vi "MPB test loop.vi"() -> ()   [LabVIEW 2020]
uses:
  controls/Send Commands.ctl
  src/Main/MPB/controls/MPB Status.ctl
  <vilib>/AKKA/PROVEtech-RBS/PROVEtechRBS.lvlib
panel:
  out "MPB Status":T1 {"InletDCportNegLowRes (VDCportNeg)" format="%.2f"; "HeatgActv (HVIL FB)" format="%.2f"; "InletACportEgy (ACfuseNeg)" format="%.2f"; "InletDCportPosLowRes (VDCportPos)" format="%.2f"; "InletACportFuseLowRes (ACfusePos)" format="%.2f"; "DCbusVoltgUpprHalf" format="%.2f"; "Vac" format="%.2f"; "TrfmrTemp2" format="%.2f"; "TrfmrTemp1" format="%.2f"; "HAPSFltCode" format="%.2f"; "ACCurr4" format="%.2f"; "ACCurr3" format="%.2f"; "ACCurr2" format="%.2f"; "ACCurr1" format="%.2f"; "HAPSCurr" format="%.2f"; "HAPSFltFlag" format="%.2f"; "HAPSVoltgOut" format="%.2f"; "HwFltCode" format="%.2f"; "HwFltFlag" format="%.2f"; "HAPSVoltgIn" format="%.2f"; "BattPortPosFuseLowRes" format="%.2f"; "BattPortNegFuseLowRes" format="%.2f"; "BattPortVoltgLowRes" format="%.2f"; "DCbusVoltg" format="%.2f"; "DCbusVoltgLowrHalf" format="%.2f"; "InletDCportVoltgHiRes" format="%.2f"; "BattPortPower" format="%.2f"; "BattVoltgHiRes" format="%.2f"; "BattCurrDAB2" format="%.2f"; "BattCurrDAB1" format="%.2f"}
  in  "Send Commands":T2
  in  "stop":bool
  # "Other"
  # "AC Port Info"
  # "Battery Port Info"
  # "Fault Info"
  # "1"
  # "2"
  # "3"
  # "4"
  # "5"
  # "6"
  # "7"
  # "DC Bus Info"
  # "HAPS Info"
  # "Temps"
  # "1"
  # "2"
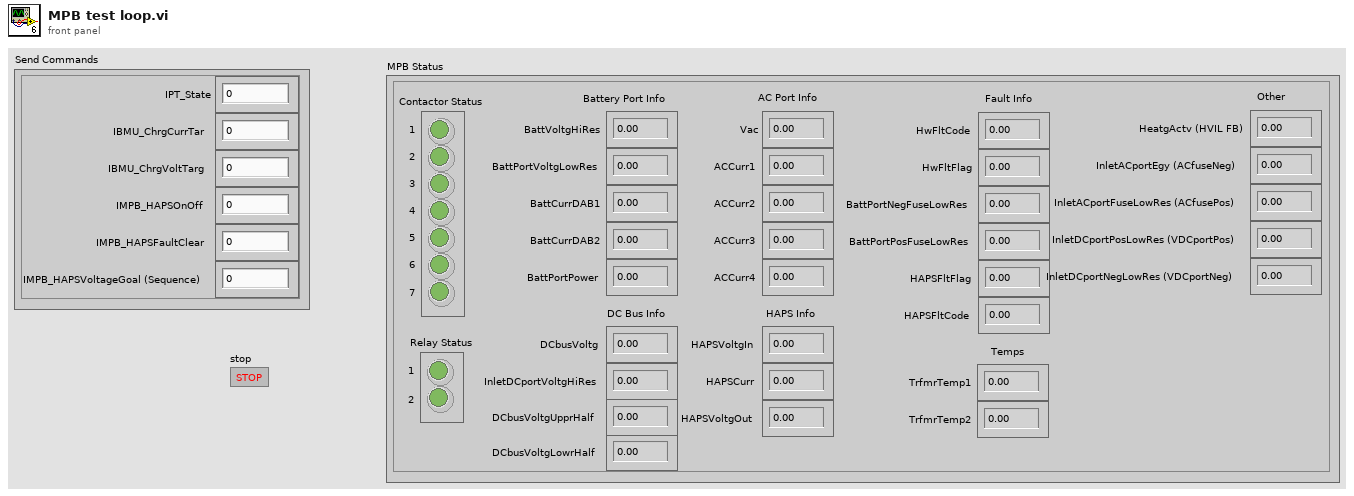
[diagram p1: front panel]
types:
  T1 = typedef "MPB Status.ctl" = cluster{"Contactor Status":bool[], "Relay Status":bool[], "BattCurrDAB1":dbl, "BattCurrDAB2":dbl, "BattVoltgHiRes":dbl, "BattPortPower":dbl, "InletDCportVoltgHiRes":dbl, "DCbusVoltgLowrHalf":dbl, "DCbusVoltg":dbl, "BattPortVoltgLowRes":dbl, "BattPortNegFuseLowRes":dbl, "BattPortPosFuseLowRes":dbl, "HAPSVoltgIn":dbl, "HwFltFlag":dbl, "HwFltCode":dbl, "HAPSVoltgOut":dbl, "HAPSFltFlag":dbl, "HAPSCurr":dbl, "ACCurr1":dbl, "ACCurr2":dbl, "ACCurr3":dbl, "ACCurr4":dbl, "HAPSFltCode":dbl, "TrfmrTemp1":dbl, "TrfmrTemp2":dbl, "Vac":dbl, "DCbusVoltgUpprHalf":dbl, "InletACportFuseLowRes (ACfusePos)":dbl, "InletDCportPosLowRes (VDCportPos)":dbl, "InletACportEgy (ACfuseNeg)":dbl, "HeatgActv (HVIL FB)":dbl, "InletDCportNegLowRes (VDCportNeg)":dbl}
  T2 = typedef "Send Commands.ctl" = cluster{"IPT_State":dbl, "IBMU_ChrgCurrTar":dbl, "IBMU_ChrgVoltTarg":dbl, "IMPB_HAPSOnOff":dbl, "IMPB_HAPSFaultClear":dbl, "IMPB_HAPSVoltageGoal (Sequence)":dbl}
  T3 = typedef "PROVEtechRBS.lvlib/RBS Session.ctl" = cluster{"core":T4, "core VI reference":refnum<vi>}
  T4 = typedef "PROVEtechRBS.lvlib/RBS Core Data.ctl" = cluster{"RBS config file":path, "RBSVeristand path":path, "TX signals":cluster{"names":string[], "values":dbl[]}, "RX signals":cluster{"names":string[], "values":dbl[]}, "TX_enable signals":cluster{"names":string[], "indices":i32[]}, "core comm":cluster{"TX":refnum<data-value>, "RX":refnum<data-value>, "status":refnum<data-value>}, "Write to System Log?":bool}
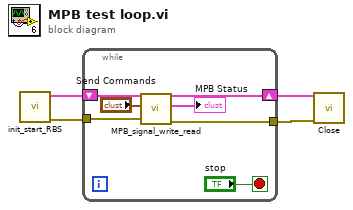
[diagram p0: block diagram]
diagram:
  n1 = call "init_start_RBS.vi"() -> ("error out"=w3:errorcluster, "RBS session out"=w4:T3)  [unwired: 10 in]
  n2 = while {
    shift-right: [w9] -> w2
    shift-left: w4 -> [w11]
    tunnel: w3 -> [w10]
    tunnel: [w8] -> w1
    stop <- "stop" stop-if-true
    n3 = call "MPB_signal_write_read.vi"("error in"=w10, "Send Commands"="Send Commands", "RBS session in"=w11) -> ("error out"=w8:errorcluster, "MPB Status"=→"MPB Status":T1, "RBS session out"=w9:T3)  [unwired: 6 in]
  }
  n4 = call <vilib>:"Close.vi"("error in (no error)"=w1, "RBS session in"=w2) -> ()  [unwired: 9 in, 1 out]
